vi "Spatial Toolbox.vi"(7 "JPG":refnum<vi>, 10 "queueName":string="PV_script", 11 "Console Reference":refnum<vi>) -> ()   [LabVIEW 2022 SP3]
uses:
  <vilib>/Utility/error.llb/Trim Whitespace One-Sided.vi
  <vilib>/Platform/browser.llb/Open URL in Default Browser (string).vi
panel:
  out "Motors 2":string
  in  "Parse":bool
  out "Onshape Path":string
  out "featureName":string
  out "offsetY":i32
  out "offsetX":i32
  out "link2Length":i32
  out "link1Length":i32
  out "imageToBaseY":i32
  out "imageToBaseX":i32
  in  "Onshape":bool
  in  "Server":bool
  out "Motors":string
  out "REPL?":bool
  out "Port open":bool
  out "UDP Port":string
  out "Onshape URL":string
  out "Server URL":string
  out "Console":string
  in  "start":bool
  in  "Save":bool
  in  "Clear":bool
  # "https://github.com/PTC-Academic/SpatialToolbox-RaspberryPi"
  # "SETTINGS"
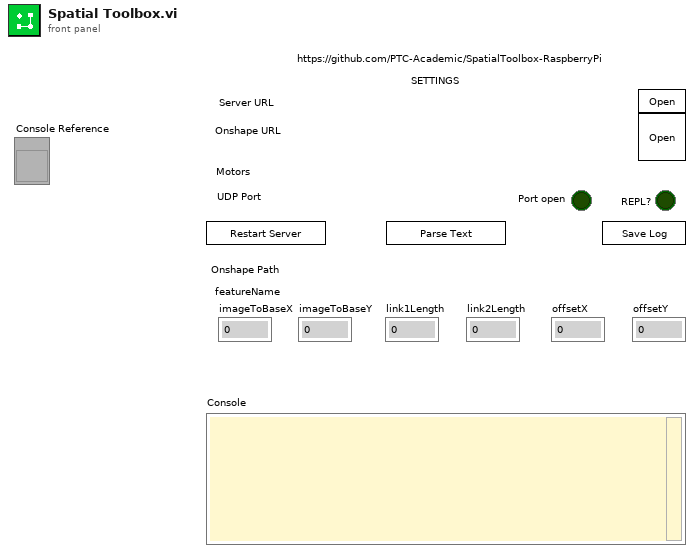
[diagram p1: front panel]
types:
  T1 = cluster{"regular expression":string, "message":string}[]
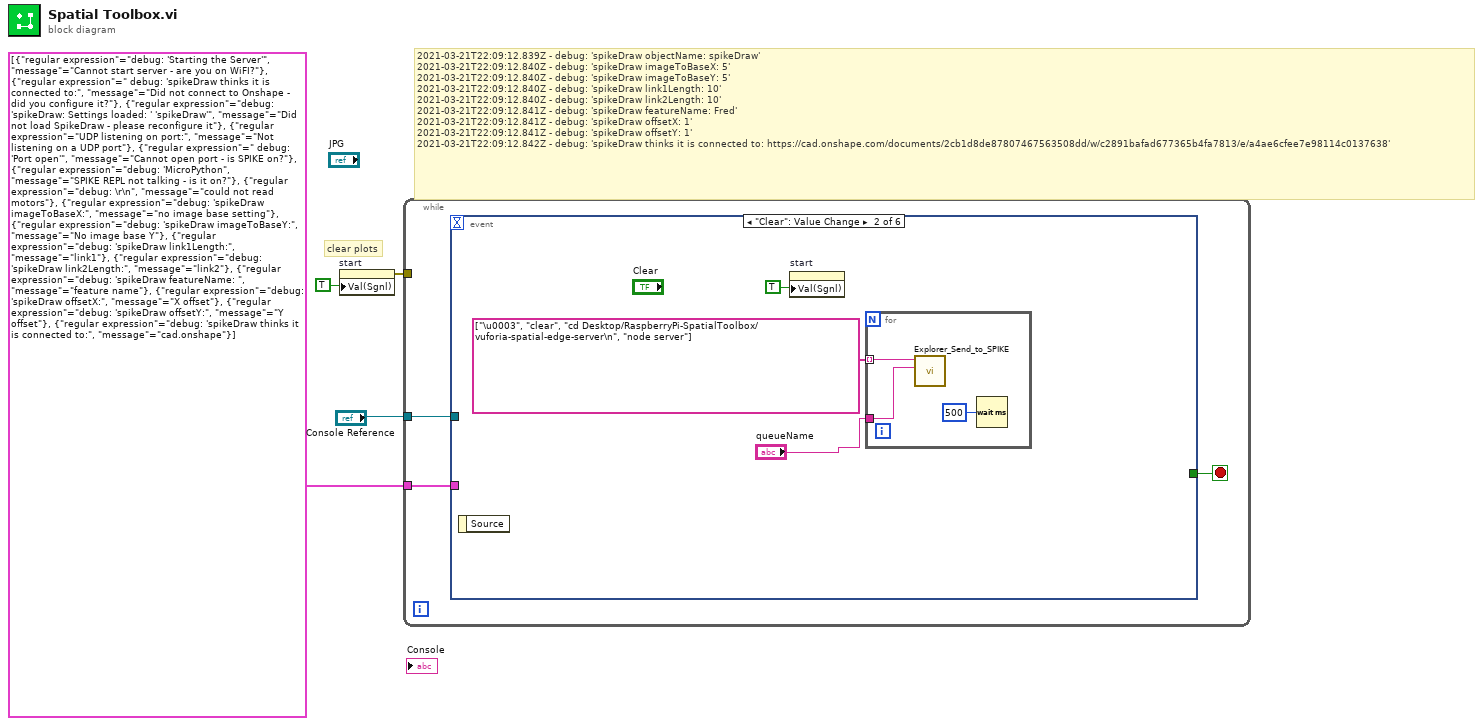
[diagram p0: block diagram]
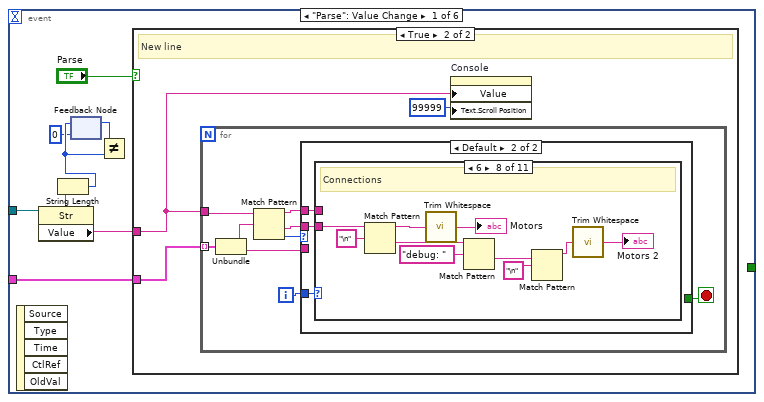
[diagram p2: hidden frame]
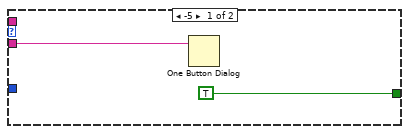
[diagram p4: hidden frame]
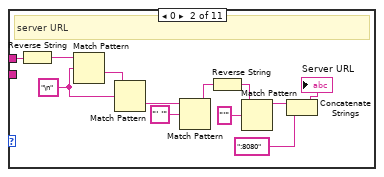
[diagram p6: hidden frame]
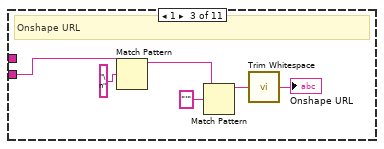
[diagram p7: hidden frame]
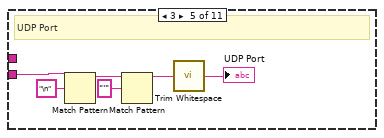
[diagram p9: hidden frame]
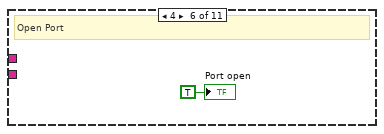
[diagram p10: hidden frame]
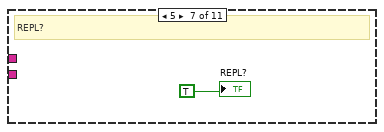
[diagram p11: hidden frame]
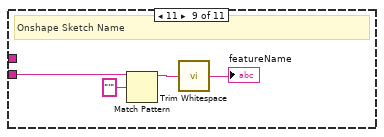
[diagram p12: hidden frame]
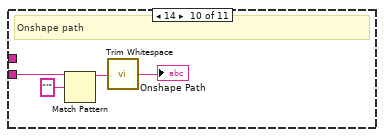
[diagram p13: hidden frame]
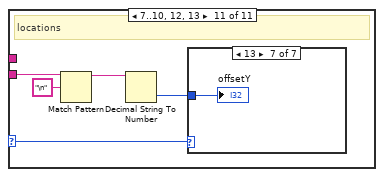
[diagram p14: hidden frame]
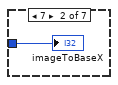
[diagram p16: hidden frame]
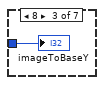
[diagram p17: hidden frame]
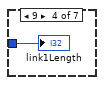
[diagram p18: hidden frame]
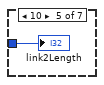
[diagram p19: hidden frame]
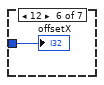
[diagram p20: hidden frame]
diagram:
  # "2021-03-21T22:09:12.839Z - debug: 'spikeDraw objectName: spikeDraw' \n2021-03-21T22:09:12.840Z - debug: 'spikeDraw imageToBaseX: 5' \n2021-03-21T22:09:12.840Z - debug: 'spikeDraw imageToBaseY: 5' \n2021-03-21T22:09:12.840Z - debug: 'spikeDraw link1Length: 10' \n2021-03-21T22:09:12.840Z - debug: 'spikeDraw link2Length: 10' \n2021-03-21T22:09:12.841Z - debug: 'spikeDraw featureName: Fred' \n2021-03-21T22:09:12.841Z - debug: 'spikeDraw offsetX: 1' \n2021-03-21T22:09:12.841Z - debug: 'spikeDraw offsetY: 1' \n2021-03-21T22:09:12.842Z - debug: 'spikeDraw thinks it is connected to: https://cad.onshape.com/documents/2cb1d8de87807467563508dd/w/c2891bafad677365b4fa7813/e/a4ae6cfee7e98114c0137638'"
  # "clear plots"
  n1 = property on="start" class="Bool (strict)"("Val(Sgnl)"=TRUE ("Value (Signaling)")) -> (error out=w1:errorcluster)  [unwired: 2 in, 1 out]
  n2 = while {
    tunnel: "Console Reference" -> [w6]
    tunnel: T1 [{"regular expression"="debug: 'Starting the Server'", "message"="Cannot start server - are you on WiFI?"}, {"regular expression"=" debug: 'spikeDraw thinks it is connected to:", "message"="Did not connect to Onshape - did you configure it?"}, {"regular expression"="debug: 'spikeDraw: Settings loaded: ' 'spikeDraw'", "message"="Did not load SpikeDraw - please reconfigure it"}, {"regular expression"="UDP listening on port:", "message"="Not listening on a UDP port"}, {"regular expression"=" debug: 'Port open'", "message"="Cannot open port - is SPIKE on?"}, {"regular expression"="debug: 'MicroPython", "message"="SPIKE REPL not talking - is it on?"}, {"regular expression"="debug: \r\n", "message"="could not read motors"}, {"regular expression"="debug: 'spikeDraw imageToBaseX:", "message"="no image base setting"}, {"regular expression"="debug: 'spikeDraw imageToBaseY:", "message"="No image base Y"}, {"regular expression"="debug: 'spikeDraw link1Length:", "message"="link1"}, {"regular expression"="debug: 'spikeDraw link2Length:", "message"="link2"}, {"regular expression"="debug: 'spikeDraw featureName: ", "message"="feature name"}, {"regular expression"="debug: 'spikeDraw offsetX:", "message"="X offset"}, {"regular expression"="debug: 'spikeDraw offsetY:", "message"="Y offset"}, {"regular expression"="debug: 'spikeDraw thinks it is connected to:", "message"="cad.onshape"}] -> [w5]
    tunnel: w1 -> [_]
    stop <- w7 stop-if-true
    n3 = event shown="[1] \"Clear\": Value Change" {
      selector: _ -> [_ _ _ _ _ _]
      dyn-events: _ -> [_ _ _ _ _ _]
      timeout: _ -> [_ _ _ _ _ _]
      tunnel: [_ _ _ _ _ w104] -> w7
      tunnel: w6 -> [w13 _ _ _ _ _]
      tunnel: w5 -> [w14 _ _ _ _ _]
      event "Parse": Value Change {
        n4 = event-data() -> ()  [unwired: 1 in, 5 out]
        n5 = property class="Str"(reference=w13) -> ("Value"=w12:string)  [unwired: 1 in, 2 out]
        n6 = String Length(string=w12) -> (length=w11:i32)
        n7 = feedback-in #1(w11) -> ()
        n8 = feedback #1(0) -> (w10:i32)
        n9 = Not Equal?(x=w10, y=w11) -> ()  [unwired: 1 out]
        n10 = case shown="True" "Parse" {
          tunnel: w12 -> [_ w15]
          tunnel: w14 -> [_ w17]
          frame False {
            # "nothing new"
          }
          frame True {
            # "New line"
            n11 = for {
              tunnel: w15 -> [w24]
              tunnel: w17 -> [w23] mode=indexing
              i -> [w20]
              stop <- w18 stop-if-true
              n12 = Unbundle(w23) -> ("regular expression"=w22:string, "message"=w21:string)
              n13 = Match Pattern(string=w24, regular expression=w22) -> (before substring=w26:string, after substring=w19:string, offset past match=w25:i32)  [unwired: 1 in, 1 out]
              n14 = case shown="Default" w25 {
                tunnel: w26 -> [_ w31]
                tunnel: w21 -> [w28 _]
                tunnel: w20 -> [_ w30]
                tunnel: w19 -> [_ w29]
                tunnel: [TRUE _] -> w18
                frame -5 {
                  n15 = One Button Dialog(message=w28) -> ()  [unwired: 1 in, 1 out]
                }
                frame Default {
                  n16 = case shown="6" w30 {
                    selector: w30 -> [_ _ _ _ _ _ _ _ _ _ w76]
                    tunnel: w31 -> [_ w43 _ _ _ _ _ _ _ _ _]
                    tunnel: w29 -> [_ _ w45 _ w51 _ _ w65 w69 w73 w79]
                    frame Default {
                    }
                    frame 0 {
                      w35 = "\n" ("regular expression")
                      # "server URL"
                      n17 = Reverse String(1:w43) -> (0:w42:string)
                      n18 = Match Pattern(string=w42, regular expression=w35) -> (after substring=w41:string)  [unwired: 1 in, 3 out]
                      n19 = Match Pattern(string=w41, regular expression=w35) -> (before substring=w39:string)  [unwired: 1 in, 3 out]
                      n20 = Match Pattern(string=w39, regular expression="' '") -> (before substring=w38:string)  [unwired: 1 in, 3 out]
                      n21 = Reverse String(1:w38) -> (0:w36:string)
                      n22 = Match Pattern(string=w36, regular expression="'") -> (before substring=w34:string)  [unwired: 1 in, 3 out]
                      n23 = Concatenate Strings(w34, ":8080" ("string")) -> (→"Server URL":string)
                    }
                    frame 1 {
                      # "Onshape URL"
                      n24 = Match Pattern(string=w45, regular expression="\n") -> (before substring=w48:string)  [unwired: 1 in, 3 out]
                      n25 = Match Pattern(string=w48, regular expression="'") -> (before substring=w49:string)  [unwired: 1 in, 3 out]
                      n26 = call <vilib>:"Trim Whitespace.vi"("string"=w49) -> ("trimmed string"=→"Onshape URL":string)  [unwired: 1 in]
                    }
                    frame 2 {
                      # "Loaded SpikeDraw?"
                    }
                    frame 3 {
                      # "UDP Port"
                      n27 = Match Pattern(string=w51, regular expression="\n") -> (before substring=w54:string)  [unwired: 1 in, 3 out]
                      n28 = Match Pattern(string=w54, regular expression="'") -> (before substring=w55:string)  [unwired: 1 in, 3 out]
                      n29 = call <vilib>:"Trim Whitespace.vi"("string"=w55) -> ("trimmed string"=→"UDP Port":string)  [unwired: 1 in]
                    }
                    frame 4 {
                      # "Open Port"
                      "Port open" <- TRUE ("Port open")
                    }
                    frame 5 {
                      # "REPL?"
                      "REPL?" <- TRUE ("Port open")
                    }
                    frame 6 {
                      # "Connections"
                      n30 = Match Pattern(string=w65, regular expression="\n") -> (before substring=w58:string, after substring=w60:string)  [unwired: 1 in, 2 out]
                      n31 = call <vilib>:"Trim Whitespace.vi"("string"=w58) -> ("trimmed string"=→"Motors":string)  [unwired: 1 in]
                      n32 = Match Pattern(string=w60, regular expression="debug: ") -> (after substring=w59:string)  [unwired: 1 in, 3 out]
                      n33 = Match Pattern(string=w59, regular expression="\n") -> (before substring=w61:string)  [unwired: 1 in, 3 out]
                      n34 = call <vilib>:"Trim Whitespace.vi"("string"=w61) -> ("trimmed string"=→"Motors 2":string)  [unwired: 1 in]
                    }
                    frame 11 {
                      # "Onshape Sketch Name"
                      n35 = Match Pattern(string=w69, regular expression="'") -> (before substring=w68:string)  [unwired: 1 in, 3 out]
                      n36 = call <vilib>:"Trim Whitespace.vi"("string"=w68) -> ("trimmed string"=→"featureName":string)  [unwired: 1 in]
                    }
                    frame 14 {
                      # "Onshape path"
                      n37 = Match Pattern(string=w73, regular expression="'") -> (before substring=w72:string)  [unwired: 1 in, 3 out]
                      n38 = call <vilib>:"Trim Whitespace.vi"("string"=w72) -> ("trimmed string"=→"Onshape Path":string)  [unwired: 1 in]
                    }
                    frame 7..10, 12, 13 {
                      # "locations"
                      n39 = Match Pattern(string=w79, regular expression="\n") -> (before substring=w78:string)  [unwired: 1 in, 3 out]
                      n40 = Decimal String To Number(string=w78) -> (number=w77:i32)  [unwired: 2 in, 1 out]
                      n41 = case shown="13" w76 {
                        tunnel: w77 -> [_ w81 w82 w83 w84 w85 w86]
                        frame 0, Default {
                        }
                        frame 7 {
                          "imageToBaseX" <- w81
                        }
                        frame 8 {
                          "imageToBaseY" <- w82
                        }
                        frame 9 {
                          "link1Length" <- w83
                        }
                        frame 10 {
                          "link2Length" <- w84
                        }
                        frame 12 {
                          "offsetX" <- w85
                        }
                        frame 13 {
                          "offsetY" <- w86
                        }
                      }
                    }
                  }
                }
              }
            }
            n42 = property on="Console" class="Str"("Value"=w15, "Text.Scroll Position"=u32 99999 ("Text.Selection:End")) -> ()  [unwired: 2 in, 2 out]
          }
        }
      }
      event "Clear": Value Change {
        n43 = event-data() -> ()  [unwired: 1 in, 1 out]
        n44 = property on="start" class="Bool (strict)"("Val(Sgnl)"=TRUE ("Value (Signaling)")) -> ()  [unwired: 2 in, 2 out]
        n45 = for {
          tunnel: string[] ["\u0003", "clear", "cd Desktop/RaspberryPi-SpatialToolbox/vuforia-spatial-edge-server\n", "node server"] -> [w92] mode=indexing
          tunnel: "queueName" -> [w90]
          n46 = call "Explorer_Send_to_SPIKE.vi"("queueName"=w90, "python"=w92) -> ()  [unwired: 9 in, 1 out]
          n47 = Wait (ms)(milliseconds to wait=u32 500) -> ()  [unwired: 1 out]
        }
      }
      event "start": Value Change {
        w93 = 0 ("imageToBaseX")
        w95 = FALSE ("REPL?")
        w94 = ""
        n48 = event-data() -> ()  [unwired: 1 in, 1 out]
        n49 = local write "imageToBaseX"(w93) -> ()
        n50 = local write "imageToBaseY"(w93) -> ()
        n51 = local write "link2Length"(w93) -> ()
        n52 = local write "link1Length"(w93) -> ()
        n53 = local write "offsetY"(w93) -> ()
        n54 = local write "offsetX"(w93) -> ()
        n55 = local write "Onshape URL"(w94) -> ()
        n56 = local write "Server URL"(w94) -> ()
        n57 = local write "Port open"(w95) -> ()
        n58 = local write "UDP Port"(w94) -> ()
        n59 = local write "Motors"(w94) -> ()
        n60 = local write "REPL?"(w95) -> ()
        n61 = local write "Motors 2"(w94) -> ()
        n62 = local write "Onshape Path"(w94) -> ()
        n63 = local write "featureName"(w94) -> ()
        n64 = local write "Console"(w94) -> ()
      }
      event "Server", "Onshape": Value Change {
        n65 = event-data() -> ()  [unwired: 1 in, 5 out]
        n66 = case shown="True" "Onshape" {
          tunnel: [w98 w99] -> w96
          frame False {
            n67 = local read "Server URL"() -> (w98:string)
          }
          frame True {
            n68 = local read "Onshape URL"() -> (w99:string)
          }
        }
        n69 = call-poly <vilib>:"Open URL in Default Browser.vi"("URL"=w96) -> ()  [unwired: 5 in, 2 out]
      }
      event "Save": Value Change {
        n70 = event-data() -> ()  [unwired: 1 in, 1 out]
        n71 = call "File Dialog"() -> ("selected path"=w101:path, "error out"=w100:errorcluster)  [unwired: 12 in, 2 out]
        n72 = case shown="No Error" w100 {
          tunnel: w101 -> [w103 _]
          frame No Error {
            n73 = local read "Console"() -> (w102:string)
            n74 = Write to Text File(file (use dialog)=w103, text=w102) -> ()  [unwired: 2 in, 3 out]
          }
          frame Error {
          }
        }
      }
      event Panel Close? {
        w104 = TRUE ("Discard?")
        n75 = event-data() -> ()  [unwired: 1 in, 1 out]
        n76 = event-data("Discard?"=w104) -> ()  [unwired: 1 in, 1 out]
      }
    }
  }
